vi "myRIO_BRig_Host_comm_getData_2D_u16__givePath.vi"(11 "input_filePath":path) -> (2 "output_data_2D":u16[][](array[numeric]), 3 "output_I_data":bool)   [LabVIEW 2014]
uses:
  <vilib>/Utility/file.llb/Read From Spreadsheet File (I64).vi
panel:
  out "error out":errorcluster
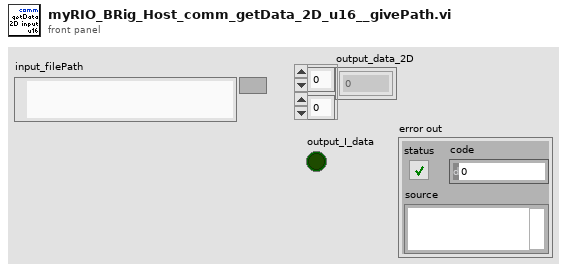
[diagram p1: front panel]
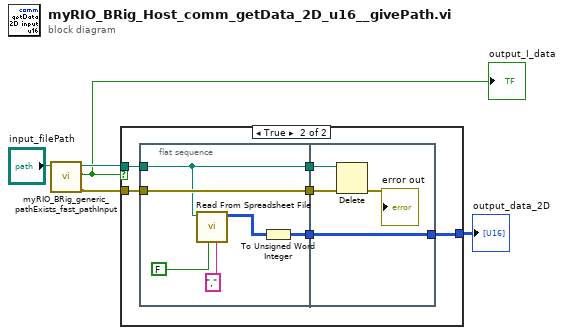
[diagram p0: block diagram]
diagram:
  n1 = call "myRIO_BRig_generic_pathExists_fast_pathInput.vi"("input_filePath"="input_filePath") -> ("output_error"=w4:errorcluster, "output_Iexist"=w2:bool, "output_filePath"=w3:path)  [unwired: 8 in]
  "output_I_data" <- w2
  n2 = case shown="True" w2 {
    tunnel: w3 -> [_ w11]
    tunnel: w4 -> [_ w8]
    tunnel: [_ w6] -> w5
    frame False {
    }
    frame True {
      n3 = flat-sequence {
        tunnel: w11 -> [w15]
        tunnel: [w15] -> w10
        tunnel: w8 -> [w17]
        tunnel: [w17] -> w9
        tunnel: [w13] -> w7
        tunnel: w10 -> [w21]
        tunnel: w9 -> [w20]
        tunnel: [w18] -> w6
        tunnel: w7 -> [w18]
        frame #0 {
          n4 = call-poly <vilib>:"Read From Spreadsheet File.vi"("delimiter (\\t)"="," ("delimiter (\\t)"), "transpose (no:F)"=FALSE, "file path (dialog if empty)"=w15) -> ("all rows"=w12:i64[][])  [unwired: 4 in, 4 out]
          n5 = To Unsigned Word Integer(number=w12) -> (unsigned 16bit integer=w13:u16[][])
        }
        frame #1 {
          n6 = Delete(path (use dialog)=w21, error in=w20) -> (error out=→"error out":errorcluster)  [unwired: 3 in, 2 out]
        }
      }
    }
  }
  "output_data_2D" <- w5
